vi "TCPServiceInit.vi"(2 "Type":string="baxter_core_msgs/ListCameras", 3 "topic":string, 4 "callerID":string) -> (0 "Success?":bool, 1 "TCP ROS Reply":string)   [LabVIEW 2012]
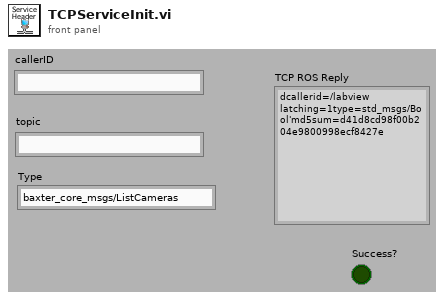
[diagram p1: front panel]
types:
  T1 = typedef "_ROSControl.ctl" = cluster{"topic port":u16, "Node":string, "topic":string, "type":string, "node port":u32, "error ":errorcluster, "Direction":T2, "APIs":string[], "Update (ms)":u16, "write queue":u16}
  T2 = typedef "_ROSDirection.ctl" = enum16{"Node", "Publisher", "Subscriber", "Service Client"}
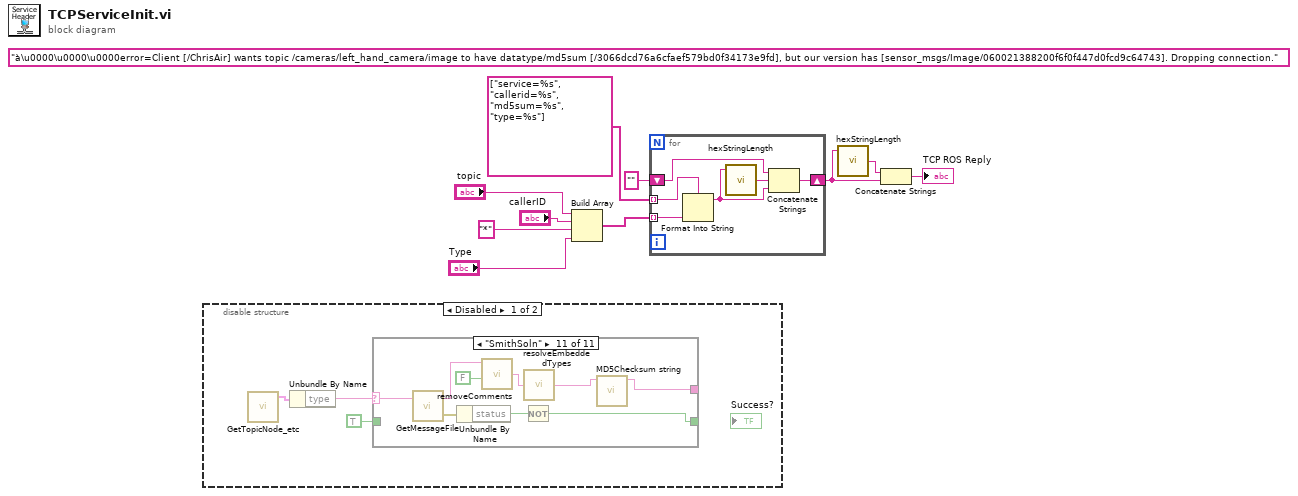
[diagram p0: block diagram]
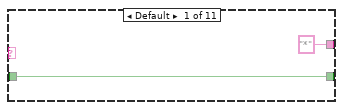
[diagram p2: hidden frame]
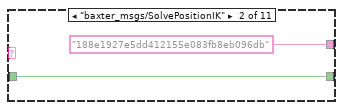
[diagram p3: hidden frame]
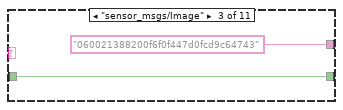
[diagram p4: hidden frame]
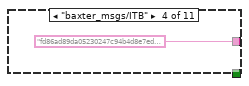
[diagram p5: hidden frame]
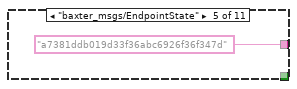
[diagram p6: hidden frame]
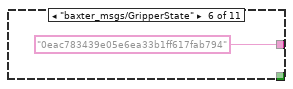
[diagram p7: hidden frame]
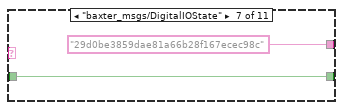
[diagram p8: hidden frame]
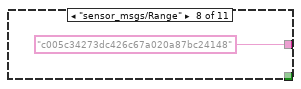
[diagram p9: hidden frame]
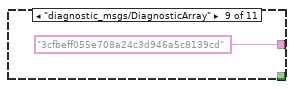
[diagram p10: hidden frame]
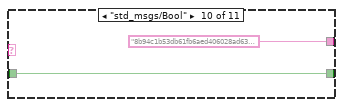
[diagram p11: hidden frame]
diagram:
  (unwired) "à\u0000\u0000\u0000error=Client [/ChrisAir] wants topic /cameras/left_hand_camera/image to have datatype/md5sum [/3066dcd76a6cfaef579bd0f34173e9fd], but our version has [sensor_msgs/Image/060021388200f6f0f447d0fcd9c64743]. Dropping connection." ("Second")
  n1 = disable-structure shown="Disabled" {
    frame Disabled {
      n2 = call "GetTopicNode_etc.vi"() -> ("ROS"=w11:T1)  [unwired: 2 in, 2 out]
      n3 = Unbundle By Name(w11) -> ("type"=w13:string)
      n4 = case shown="\"SmithSoln\"" w13 {
        selector: w13 -> [_ _ _ _ _ _ _ _ _ _ w33]
        tunnel: ["*" "188e1927e5dd412155e083fb8eb096db" "060021388200f6f0f447d0fcd9c64743" ("MD5 Sum") "fd86ad89da05230247c94b4d8e7ed306" ("MD5 Sum") "a7381ddb019d33f36abc6926f36f347d" ("MD5 Sum") "0eac783439e05e6ea33b1ff617fab794" ("MD5 Sum") "29d0be3859dae81a66b28f167ecec98c" ("MD5 Sum") "c005c34273dc426c67a020a87bc24148" ("Second") "3cfbeff055e708a24c3d946a5c8139cd" ("MD5 Sum") "8b94c1b53db61fb6aed406028ad6332a" ("MD5 Sum") w29] -> _
        tunnel: [w15 w16 w18 _ _ _ w23 _ _ w27 w31] -> _
        tunnel: TRUE ("status") -> [w15 w16 w18 _ _ _ w23 _ _ w27 _]
        frame Default {
        }
        frame "baxter_msgs/SolvePositionIK" {
        }
        frame "sensor_msgs/Image" {
        }
        frame "baxter_msgs/ITB" {
        }
        frame "baxter_msgs/EndpointState" {
        }
        frame "baxter_msgs/GripperState" {
        }
        frame "baxter_msgs/DigitalIOState" {
        }
        frame "sensor_msgs/Range" {
        }
        frame "diagnostic_msgs/DiagnosticArray" {
        }
        frame "std_msgs/Bool" {
        }
        frame "SmithSoln" {
          n5 = call "GetMessageFile.vi"("type"=w33) -> ("error out"=w34:errorcluster, "File"=w35:string)  [unwired: 1 in]
          n6 = Unbundle By Name(w34) -> ("status"=w32:bool)
          n7 = call "removeComments.vi"("Trim Whitespace? (F)"=FALSE ("Trim Whitespace?"), "String"=w35) -> ("Body"=w37:string)  [unwired: 2 in, 2 out]
          n8 = Not(x=w32) -> (.not. x?=w31:bool)
          n9 = call "resolveEmbeddedTypes.vi"("Message Definition"=w37) -> ("Md5 Text"=w30:string)
          n10 = call <vilib>:"MD5Checksum string.vi"("Message String"=w30) -> ("MD5 message-digest"=w29:string)  [unwired: 10 in]
        }
      }
    }
    frame Enabled {
    }
  }
  n11 = Build Array("topic", "callerID", "*", "Type") -> (w5:string[])
  n12 = for {
    tunnel: w5 -> [w42] mode=indexing
    tunnel: string[] ["service=%s", "callerid=%s", "md5sum=%s", "type=%s"] -> [w43] mode=indexing
    shift-right: [w38] -> w10
    shift-left: "" -> [w39]
    n13 = Format Into String(format string=w43, w42) -> (resulting string=w40:string)  [unwired: 2 in, 1 out]
    n14 = call "hexStringLength.vi"("String"=w40) -> ("String hex length"=w41:string)  [unwired: 2 in]
    n15 = Concatenate Strings(w39, w41, w40) -> (w38:string)
  }
  n16 = call "hexStringLength.vi"("String"=w10) -> ("String hex length"=w7:string)  [unwired: 2 in]
  n17 = Concatenate Strings(w7, w10) -> (→"TCP ROS Reply":string)
